vi "LVProjectShortcut_GetItemIcon.vi"(8 "error in (no error)":errorcluster, 10 "File Path":path) -> (0 "error out":errorcluster, 2 "Icon Path":path)   [LabVIEW 2017]
uses:
  <vilib>/Utility/lvfile.llb/FT_FileTypes.ctl
  <vilib>/Utility/lvfile.llb/NI_FileType.lvlib
panel:
  out "file type":T1
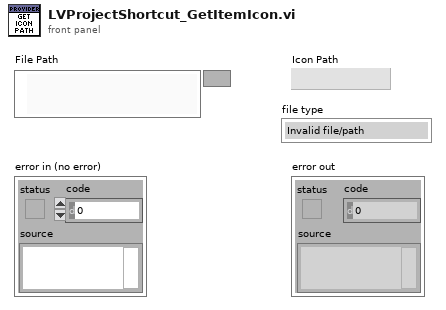
[diagram p1: front panel]
types:
  T1 = typedef "NI_FileType.lvlib/FT_FileTypes.ctl" = enum32{"Invalid file/path", "Unknown type", "Instrument", "Control", "Polymorphic VI", "Project", "Library", "LVClass", "XControl", "XNode", "CIN", "Run-time menu", "Palette menu", "LLB", "Shortcut", "Directory", "Class Private Data Control", "Statechart", "MathScript .m file", "Ladder Diagram", "LVLibp"}
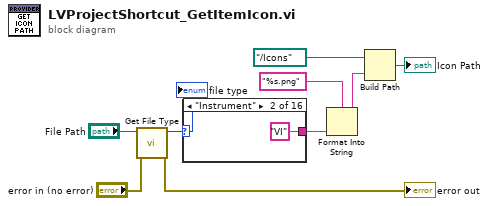
[diagram p0: block diagram]
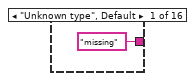
[diagram p2: hidden frame]
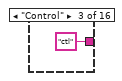
[diagram p3: hidden frame]
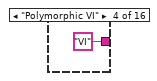
[diagram p4: hidden frame]
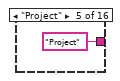
[diagram p5: hidden frame]
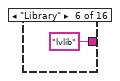
[diagram p6: hidden frame]
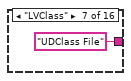
[diagram p7: hidden frame]
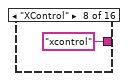
[diagram p8: hidden frame]
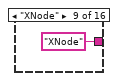
[diagram p9: hidden frame]
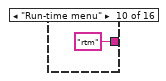
[diagram p10: hidden frame]
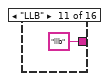
[diagram p11: hidden frame]
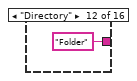
[diagram p12: hidden frame]
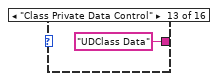
[diagram p13: hidden frame]
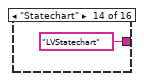
[diagram p14: hidden frame]
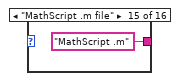
[diagram p15: hidden frame]
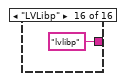
[diagram p16: hidden frame]
diagram:
  n1 = call <vilib>:"Get File Type.vi"("error in (no error)"="error in (no error)", "path"="File Path") -> ("error out"=→"error out":errorcluster, "file type"=w4:T1)  [unwired: 7 in, 1 out]
  "file type" <- w4
  n2 = case shown="\"Instrument\"" w4 {
    tunnel: ["missing" "VI" "ctl" "VI" "Project" "lvlib" "UDClass File" "xcontrol" "XNode" "rtm" "llb" "Folder" "UDClass Data" "LVStatechart" "MathScript .m" "lvlibp"] -> w3
    frame "Unknown type", Default {
    }
    frame "Instrument" {
    }
    frame "Control" {
    }
    frame "Polymorphic VI" {
    }
    frame "Project" {
    }
    frame "Library" {
    }
    frame "LVClass" {
    }
    frame "XControl" {
    }
    frame "XNode" {
    }
    frame "Run-time menu" {
    }
    frame "LLB" {
    }
    frame "Directory" {
    }
    frame "Class Private Data Control" {
    }
    frame "Statechart" {
    }
    frame "MathScript .m file" {
    }
    frame "LVLibp" {
    }
  }
  n3 = Format Into String(format string="%s.png", w3) -> (resulting string=w7:string)  [unwired: 2 in, 1 out]
  n4 = Build Path(base path=path "../Icons" ("Icon Path"), name or relative path=w7) -> (appended path=→"Icon Path":path)
